vi "Generate Boolean Array SubVI.vi"(8 "Activate: 1\nDeactivate: 0":bool, 11 "Tube":u8) -> (3 "Boolean array":bool[](array[boolean]))   [LabVIEW 2020]
panel:
  # "___"
  # "___"
  # "___"
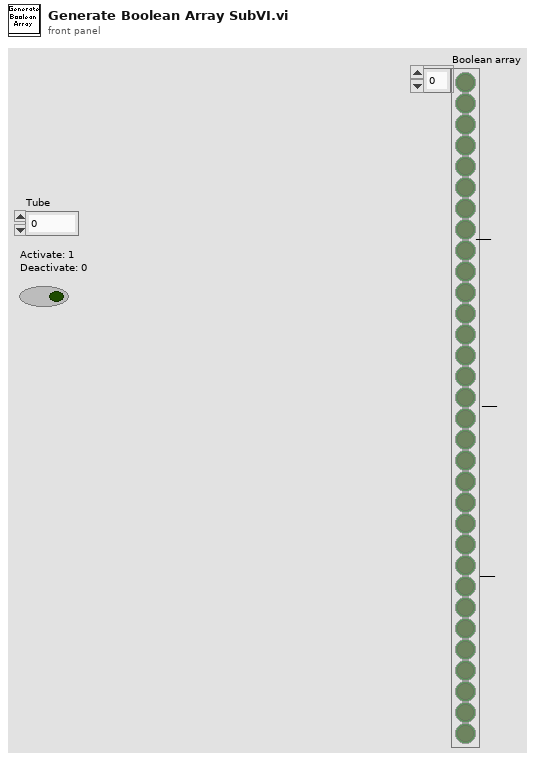
[diagram p1: front panel]
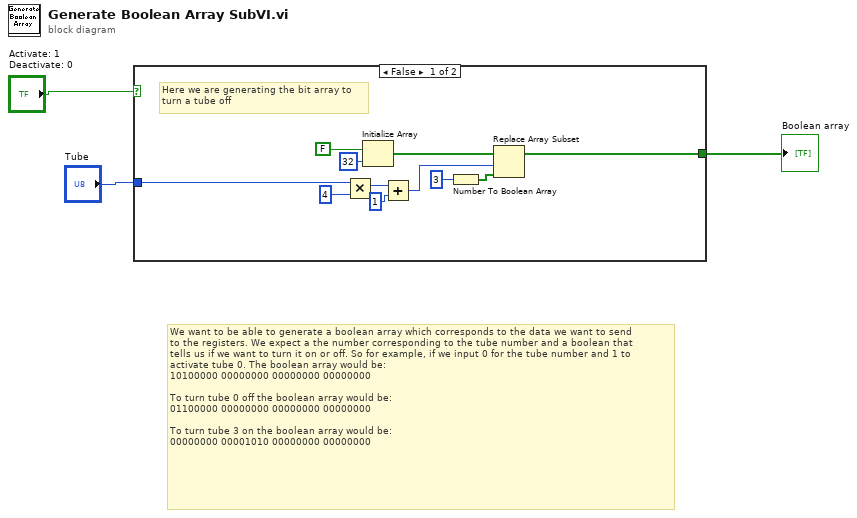
[diagram p0: block diagram]
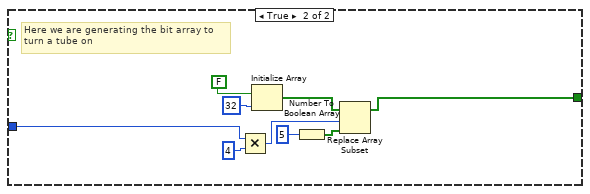
[diagram p2: hidden frame]
diagram:
  # "We want to be able to generate a boolean array which corresponds to the data we want to send \nto the registers. We expect a the number corresponding to the tube number and a boolean that\ntells us if we want to turn it on or off. So for example, if we input 0 for the tube number and 1 to\nactivate tube 0. The boolean array would be:\n10100000 00000000 00000000 00000000 \n\nTo turn tube 0 off the boolean array would be:\n01100000 00000000 00000000 00000000\n\nTo turn tube 3 on the boolean array would be:\n00000000 00001010 00000000 00000000"
  n1 = case shown="False" "Activate: 1\nDeactivate: 0" {
    tunnel: "Tube" -> [w9 w16]
    tunnel: [w8 w15] -> w1
    frame False {
      # "Here we are generating the bit array to \nturn a tube off"
      n2 = Multiply(x=w9, y=4) -> (x*y=w5:i32)
      n3 = Initialize Array(FALSE, 32) -> (w10:bool[])
      n4 = Add(x=w5, y=1) -> (x+y=w6:i32)
      n5 = Number To Boolean Array(number=3) -> (Boolean array=w13:bool[])
      n6 = Replace Array Subset(array=w10, new element=w13, index=w6) -> (w8:bool[])
    }
    frame True {
      # "Here we are generating the bit array to \nturn a tube on"
      n7 = Multiply(x=w16, y=4) -> (x*y=w18:i32)
      n8 = Initialize Array(FALSE, 32) -> (w21:bool[])
      n9 = Number To Boolean Array(number=5) -> (Boolean array=w17:bool[])
      n10 = Replace Array Subset(array=w21, new element=w17, index=w18) -> (w15:bool[])
    }
  }
  "Boolean array" <- w1
